vi "SLSC Get SLSC Chassis Address in Host.vi"(8 "error in (no error)":errorcluster, 11 "Parent Ref":T1 format="%.0x") -> (0 "error out":errorcluster, 1 "ChassisIDType":i32(ring) items=["ChassisName", "HostnameIPAddress"], 2 "IP Address":string, 3 "Item Ref out":T1 format="%.0x")   [LabVIEW 2017, in "SLSC CD System Explorer.lvlib"]
uses:
  SLSC CD System Explorer.lvlib
  <vilib>/NI Veristand/Custom Device API/Custom Device Item Ref.ctl
  NationalInstruments.VeriStand.SystemDefinitionAPI
  <vilib>/NI VeriStand/Custom Device API/Custom Device API.lvlib
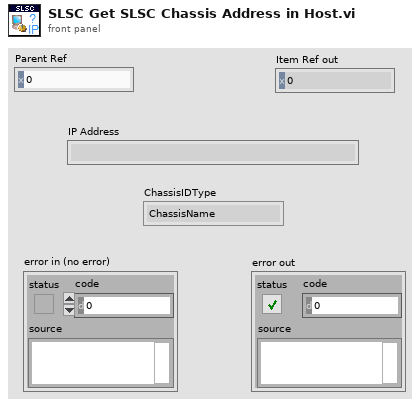
[diagram p1: front panel]
types:
  T1 = typedef "Custom Device API.lvlib/Custom Device Item Ref.ctl" = u64
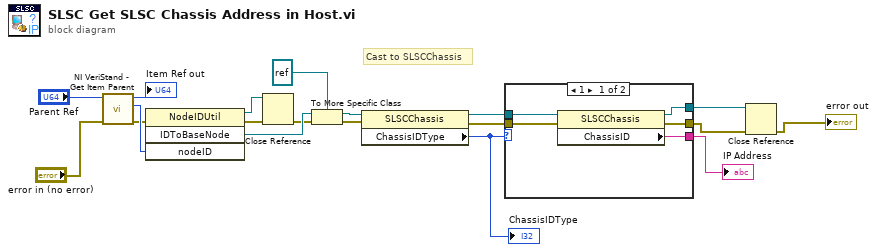
[diagram p0: block diagram]
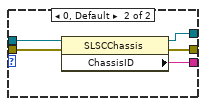
[diagram p2: hidden frame]
diagram:
  # "Cast to SLSCChassis"
  n1 = call <vilib>:"NI VeriStand - Get Item Parent.vi"("error in (no error)"="error in (no error)", "Item Ref in"="Parent Ref") -> ("error out"=w17:errorcluster, "Parent Ref"=w19:T1, "Item Ref out"=→"Item Ref out":T1)  [unwired: 6 in, 1 out]
  n2 = invoke class="NodeIDUtil" method="IDToBaseNode"(error in=w17, "nodeID"=w19) -> (reference out=w11:refnum<k24>, error out=w12:errorcluster, "IDToBaseNode"=w14:refnum<k24>)  [unwired: 2 in, 1 out]
  n3 = Close Reference(reference=w11, error in (no error)=w12) -> (error out=w13:errorcluster)
  n4 = To More Specific Class(target class=refnum<k24> refnum, reference=w14, error in=w13) -> (specific class reference=w8:refnum<k24>, error out=w7:errorcluster)
  n5 = property class="SLSCChassis"(reference=w8, error in=w7) -> (reference out=w6:refnum<k24>, error out=w5:errorcluster, "ChassisIDType"=w2:i32)
  "ChassisIDType" <- w2
  n6 = case shown="1" w2 {
    tunnel: [w24 w29] -> w16
    tunnel: w6 -> [w23 w28]
    tunnel: w5 -> [w22 w27]
    tunnel: [w21 w26] -> w4
    tunnel: [w20 w25] -> w3
    frame 1 {
      n7 = property class="SLSCChassis"(reference=w23, error in=w22) -> (reference out=w21:refnum<k24>, error out=w20:errorcluster, "ChassisID"=w24:string)
    }
    frame 0, Default {
      n8 = property class="SLSCChassis"(reference=w28, error in=w27) -> (reference out=w26:refnum<k24>, error out=w25:errorcluster, "ChassisID"=w29:string)
    }
  }
  "IP Address" <- w16
  n9 = Close Reference(reference=w4, error in (no error)=w3) -> (error out=→"error out":errorcluster)
